vi "V7310.Main.Stop.vi"(8 "error in":errorcluster, 11 "Data in":T1={"Status"={"State"=enum."Init", "LaserStatus"=enum."-", "LaserStatusRaw"="", "Ref"=refnum, "RTC TS"=timestamp(0 s since 1904-01-01), "Conn TS"=timestamp(0 s since 1904-01-01), "Msg"=[], "JobInUse"="", "Jobs"=[], "Vars"=[]}, "Sets"={"Address"="192.168.2.1", "Timeout_ms"=5000, "ReconnectPeriod_s"=0, "JobInUse"="", "CoordinatesOffset"={"X"=0.0, "Y"=0.0}}}) -> (0 "error out":errorcluster, 3 "Data out":T1={"Status"={"State"=enum."Init", "LaserStatus"=enum."-", "LaserStatusRaw"="", "Ref"=refnum, "RTC TS"=timestamp(0 s since 1904-01-01), "Conn TS"=timestamp(0 s since 1904-01-01), "Msg"=[], "JobInUse"="", "Jobs"=[], "Vars"=[]}, "Sets"={"Address"="192.168.2.1", "Timeout_ms"=5000, "ReconnectPeriod_s"=0, "JobInUse"="", "CoordinatesOffset"={"X"=0.0, "Y"=0.0}}})   [LabVIEW 2016]
uses:
  V7310.Data.ctl
  V7310.Data.Status.ctl
  V7310.Data.Status.State.ctl
  LowLevel/V7310.LaserStatus.ctl
  LowLevel/V7310.Message.Data.ctl
  LowLevel/V7310.Job.Variable.ctl
  V7310.Data.Sets.ctl
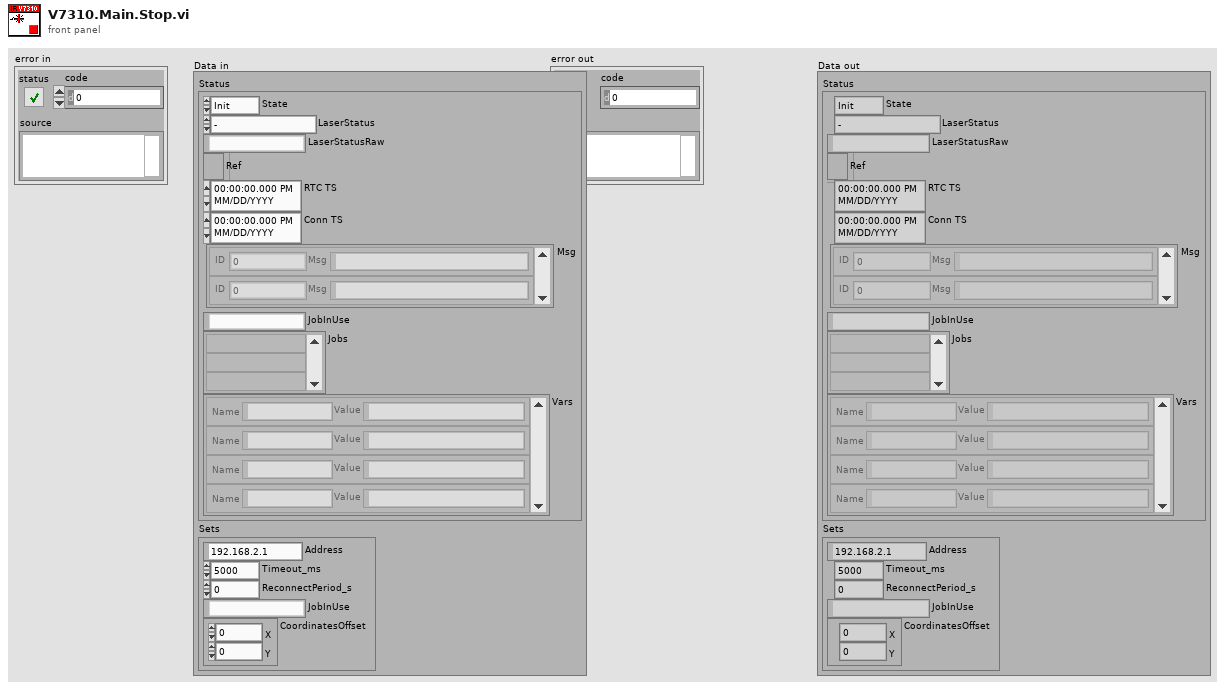
[diagram p1: front panel]
types:
  T1 = typedef "V7310.Data.ctl" = cluster{"Status":T2, "Sets":T7}
  T2 = typedef "V7310.Data.Status.ctl" = cluster{"State":T3, "LaserStatus":T4, "LaserStatusRaw":string, "Ref":refnum<k5>, "RTC TS":timestamp, "Conn TS":timestamp, "Msg":T5[], "JobInUse":string, "Jobs":string[], "Vars":T6[]}
  T3 = typedef "V7310.Data.Status.State.ctl" = enum16{"First", "Init", "Msg", "Error", "Abort", "Idle", "Run"}
  T4 = typedef "V7310.LaserStatus.ctl" = enum16{"-", "FatalError", "Initialize", "KeySwitchOpen", "TimeoutInterlock", "InterlockOpen", "StartUp", "ShutterlockOpen", "Standby", "Ready", "PrepareForMarking", "WaitForTrigger", "Marking"}
  T5 = typedef "V7310.Message.Data.ctl" = cluster{"ID":i32, "Msg":string}
  T6 = typedef "V7310.Job.Variable.ctl" = cluster{"Name":string, "Value":string}
  T7 = typedef "V7310.Data.Sets.ctl" = cluster{"Address":string, "Timeout_ms":i32, "ReconnectPeriod_s":i32, "JobInUse":string, "CoordinatesOffset":cluster{"X":dbl, "Y":dbl}}
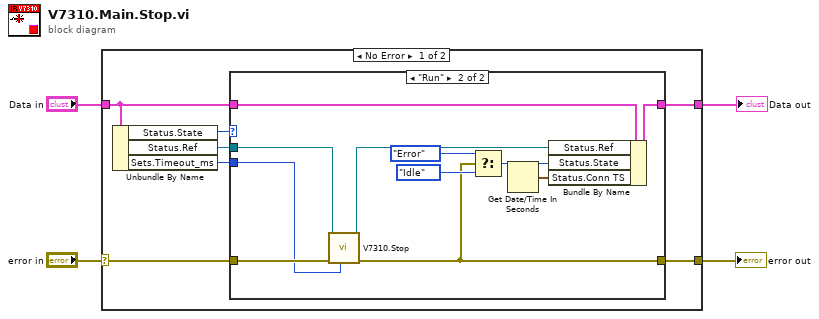
[diagram p0: block diagram]
diagram:
  n1 = case shown="No Error" "error in" {
    selector: "error in" -> [w9 w26]
    tunnel: [w7 w26] -> w3
    tunnel: "Data in" -> [w10 w25]
    tunnel: [w11 w25] -> w1
    frame No Error {
      n2 = Unbundle By Name(w10) -> ("Status.State"=w5:T3, "Status.Ref"=w6:refnum<k5>, "Sets.Timeout_ms"=w8:i32)
      n3 = case shown="\"Run\"" w5 {
        tunnel: [w13 w24] -> w11
        tunnel: w10 -> [w13 w23]
        tunnel: w9 -> [w12 w19]
        tunnel: w8 -> [_ w18]
        tunnel: [w12 w17] -> w7
        tunnel: w6 -> [_ w15]
        frame Default {
        }
        frame "Run" {
          n4 = call "V7310.Stop.vi"("timeout ms (5000)"=w18, "error in"=w19, "Connection in"=w15) -> ("error out"=w17:errorcluster, "Connection out"=w16:refnum<k5>)  [unwired: 7 in]
          n5 = Select(t=V7310.Data.Status.State."Error" ("Status.State"), s=w17, f=V7310.Data.Status.State."Idle" ("Status.State")) -> (s? t:f=w20:T3)
          n6 = Get Date/Time In Seconds() -> (seconds since 1Jan1904=w14:timestamp)
          n7 = Bundle By Name(cluster=w23, "Status.Ref"=w16, "Status.State"=w20, "Status.Conn TS"=w14) -> (w24:T1)
        }
      }
    }
    frame Error {
    }
  }
  "error out" <- w3
  "Data out" <- w1
